vi "IVtrace.vi"(0 "LINX Resource":T1, 5 "LED On":bool, 7 "Voltage Steps":i32, 9 "Rf":dbl, 11 "error in (no error)":errorcluster) -> (4 "LINX Resource 2":T1, 6 "PD Voltage":dbl[](array[numeric]), 8 "PD Current":dbl[](array[numeric]), 15 "Error Out":errorcluster)   [LabVIEW 2020]
uses:
  <vilib>/MakerHub/LINX/Private/Type Defs/LINX Ref.ctl
  <vilib>/MakerHub/LINX/Private/Type Defs/Platform.ctl
  <vilib>/MakerHub/LINX/Private/Type Defs/Interface.ctl
  <vilib>/MakerHub/LINX/Private/Device/Type Defs/LINX Device Config.ctl
  <vilib>/MakerHub/LINX/Private/Device/Type Defs/TCP Config.ctl
  <vilib>/MakerHub/LINX/Private/Device/Type Defs/Channels.ctl
  <vilib>/MakerHub/LINX/Public/Peripherals/Digital/Digital Write 1 Chan.vi
  <vilib>/MakerHub/LINX/Public/Peripherals/Digital/Digital Write N Chans.vi
  <vilib>/MakerHub/LINX/Private/Local IO/LinxDigitalWrite.vi
  <vilib>/MakerHub/LINX/Public/Utilities/Check Channel.vi
  <vilib>/MakerHub/LINX/Private/Utilties/Generate Error.vi
  <vilib>/MakerHub/LINX/LMH-LINX.lvlib
  <vilib>/MakerHub/LINX/Private/Device/Device.lvlib
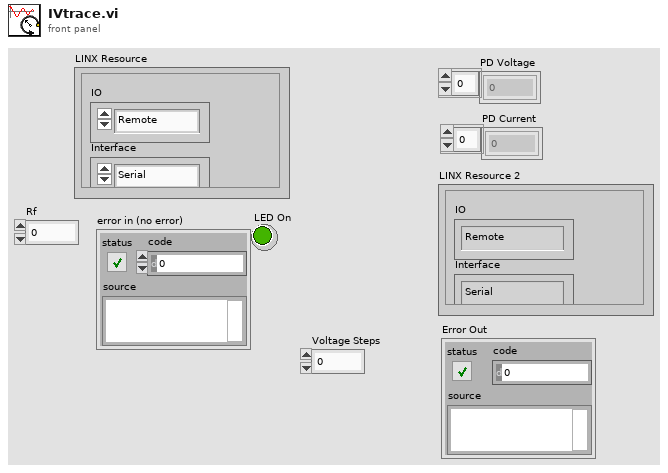
[diagram p1: front panel]
types:
  T1 = typedef "LMH-LINX.lvlib/LINX Ref.ctl" = cluster{"IO":T2, "Interface":T3, "LINX Device Config":T4}
  T2 = typedef "LMH-LINX.lvlib/Platform.ctl" = enum16{"Remote", "Local"}
  T3 = typedef "LMH-LINX.lvlib/Interface.ctl" = enum16{"Serial", "TCP"}
  T4 = typedef "LMH-LINX.lvlib/Device.lvlib/LINX Device Config.ctl" = cluster{"Interface":T3, "COM Port":refnum<visa-resource-name>, "TCP Configuration":T5, "Device Family":u8, "Device ID":u8, "Device Name":string, "TCP Ref":refnum<k5>, "Channels":T6}
  T5 = typedef "LMH-LINX.lvlib/Device.lvlib/TCP Config.ctl" = cluster{"IP Address":string, "Port":u16}
  T6 = typedef "LMH-LINX.lvlib/Channels.ctl" = cluster{"DI":u8[], "DO":u8[], "AI":u8[], "AO":u8[], "PWM":u8[], "QE":u8[], "UART":u8[], "I2C 2":u8[], "SPI":u8[], "CAN":u8[], "Servo":u8[], "AI Ref (V)":dbl, "AI Resolution (Bits)":u8, "AO Ref (V)":dbl, "AO Resolution (Bits)":u8}
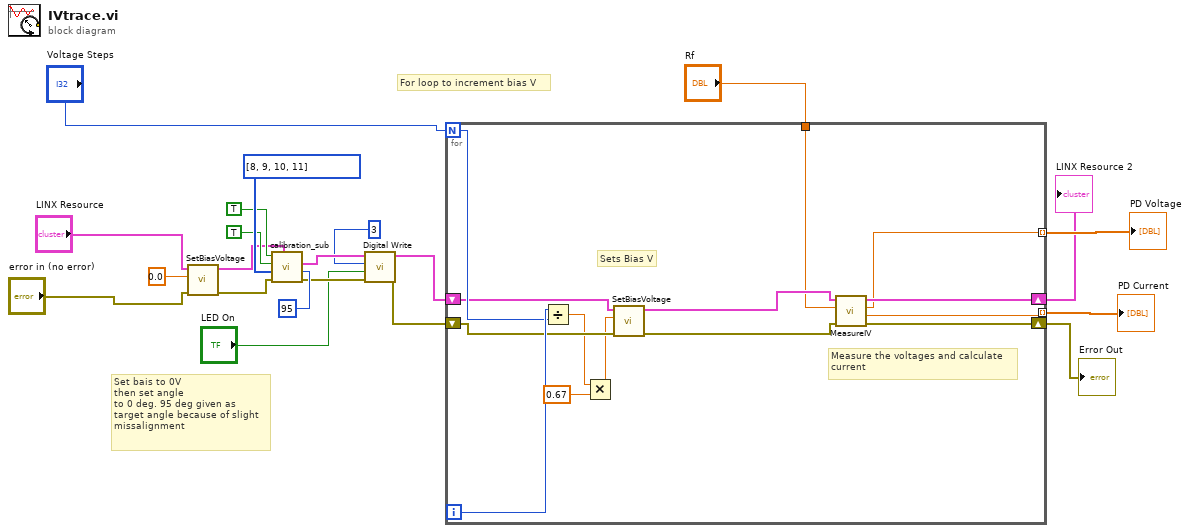
[diagram p0: block diagram]
diagram:
  # "Set bais to 0V\nthen set angle\nto 0 deg. 95 deg given as\ntarget angle because of slight\nmissalignment"
  # "For loop to increment bias V"
  n1 = call "SetBiasVoltage.vi"("Error In"="error in (no error)", "Bias V"=0.0, "LINX Resource"="LINX Resource") -> ("Error Out"=w3:errorcluster, "LINX Resource 2"=w2:T1)  [unwired: 5 in]
  n2 = call "calibration_sub.vi"("Angle in"=95, "LINX Resource"=w2, "error in (no error)"=w3, "DO Channels"=u8[] [8, 9, 10, 11], "CCW"=TRUE, "Start calibration"=TRUE) -> ("error out"=w15:errorcluster, "LINX Resource out"=w16:T1)  [unwired: 3 in, 1 out]
  n3 = call-poly <vilib>:"Digital Write.vi"("Error In"=w15, "Output Value"="LED On", "DO Channel"=u8 3, "LINX Resource"=w16) -> ("Error Out"=w14:errorcluster, "LINX Resource"=w13:T1)  [unwired: 6 in]
  n4 = for {
    N: "Voltage Steps" -> [w34]
    tunnel: [w31] -> w10 mode=indexing
    tunnel: [w30] -> w9 mode=indexing
    tunnel: "Rf" -> [w25]
    shift-right: [w33] -> w8
    shift-left: w13 -> [w29]
    shift-right: [w32] -> w7
    shift-left: w14 -> [w28]
    i -> [w35]
    # "Measure the voltages and calculate\ncurrent"
    # "Sets Bias V"
    n5 = Divide(x=w35, y=w34) -> (x/y=w24:dbl)
    n6 = Multiply(x=w24, y=0.67) -> (x*y=w23:dbl)
    n7 = call "SetBiasVoltage.vi"("Error In"=w28, "Bias V"=w23, "LINX Resource"=w29) -> ("Error Out"=w26:errorcluster, "LINX Resource 2"=w27:T1)  [unwired: 5 in]
    n8 = call "MeasureIV.vi"("Error In"=w26, "Rf"=w25, "LINX Resource"=w27) -> ("Error Out"=w32:errorcluster, "PD Current (A)"=w30:dbl, "PD Voltage (V)"=w31:dbl, "LINX Resource 2"=w33:T1)  [unwired: 5 in]
  }
  "PD Voltage" <- w10
  "PD Current" <- w9
  "LINX Resource 2" <- w8
  "Error Out" <- w7
